vi "401_Add_AuditDataToDB.vi"(0 "Str(T)/Num":bool, 2 "Activity":string, 3 "Current Value":dbl, 4 "Previous Value":dbl, 5 "Activity":T2=enum."User show functionality for Info", 6 "Enum(F)/Str":bool, 7 "error in (no error)":errorcluster, 8 "Current Value":string, 12 "Previous Value":string) -> (27 "error out":errorcluster)   [LabVIEW 2015]
uses:
  Utilities/TypeDefs/401_Audit_Activity.ctl
  <vilib>/addons/database/Connection.llb/Conn ObjectReference.ctl
  System Settings/Modules/LV2GActions.ctl
  <vilib>/addons/database/NI_Database_API.lvlib
  <vilib>/addons/database/Connection.llb/DB Tools Open Connec (String).vi
panel:
  in  "Refnum in":T1
  out "Refnum out":T1
  # "INPUT"
  # "OUTPUT"
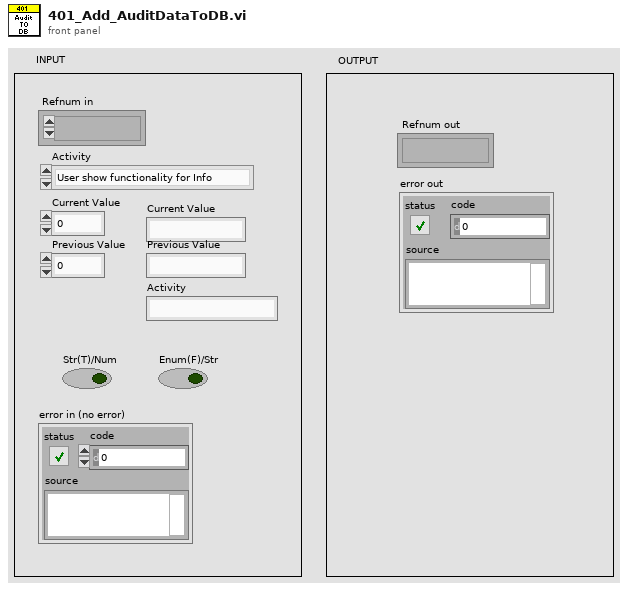
[diagram p1: front panel]
types:
  T1 = typedef "NI_Database_API.lvlib/Conn ObjectReference.ctl" = refnum<k1>
  T2 = typedef "401_Audit_Activity.ctl" = enum16{"User login sucessfully", "User login fail", "User lock", "User sign out", "User added succesfully", "User edit succesFully", "User delete succesfully", "Reset password", "Forgot Password", "User change security policy", "User change user rights", "User allowed functionality for inspection", "User allowed  functionality for recipe", "User allowed functionality for teach", "User allowed  for user management", "User allowed for camera settings", "User allowed functionality for Hardware Check", "User allowed functionality for printer settings", "User allowed functionality for server settings", "User allowed  for third party settings", "User allowed  for System settings", "User allowed functionality For Test I/O", "User allowed and show functionality For Fault Images", "User allowed functionality for Production Report", "User allowed functionality for Audit Report", "User allowed functionality for Help", "User allowed functionality for  Info", "User show functionality for Inspection", "User show functionality for Teach", "User show functionality for Recipe", "User show functionality for User Management", "User show functionality for Camera Settings", "User show functionality for Hardware Check", "User show functionality for printer Settings", "User show functionality  for Server Settings", "User show functionality for Third party Settings", "User show functionality for System settings", "User show functionality for Test I/O", "User show functionality for Fault Images", "User show functionality for Production Report", "User show functionality for Audit Report", "User show functionality for Help", "User show functionality for Info", "User update Security Policy", "User added Recipe sucessfully", "User delete Recipe sucessfully", "User rename Recipe sucessfully", "User save Camera Settings sucessfully ", "User Close with out save", "User change Brightness", "User change Exposure Time", "User change Gain Value", "User change Saturation", "User change Gamma", "User change Sharpness", "User change Hue", "User change White Balance", "User change  Comport ", "User save Test I/o settings sucessfully", "User close with out saving ", "User change Light Timing ", "User change Light Flash ", "Camera Ready", "User change Inactive Period ", "User change Grab Delay", "User change Timed Output", "User change No Of Track", "User change Output Polarity ", "User chnage Output Timing", "User change Track Output ", "User Taught sucessfully", "User close with out  Taught.", "User could not able To Add User", "User could not Delete", "User could not Updated", "User could not change Security Policy", "User could not change User Rights"}
  T3 = typedef "LV2GActions.ctl" = enum16{"Read", "Write", "Current", "Update", "UpdateSystemSettings", "UpdateModel"}
  T4 = cluster{"UserName":string, "Group Level":u16, "Theme":u16, "Software Type":u16, "System Language":u16, "Master":bool, "Recipe":string, "Batch":string, "Simulate":bool, "Trigger Activation":u16, "DateFormat":u16, "HardwareTest":bool}
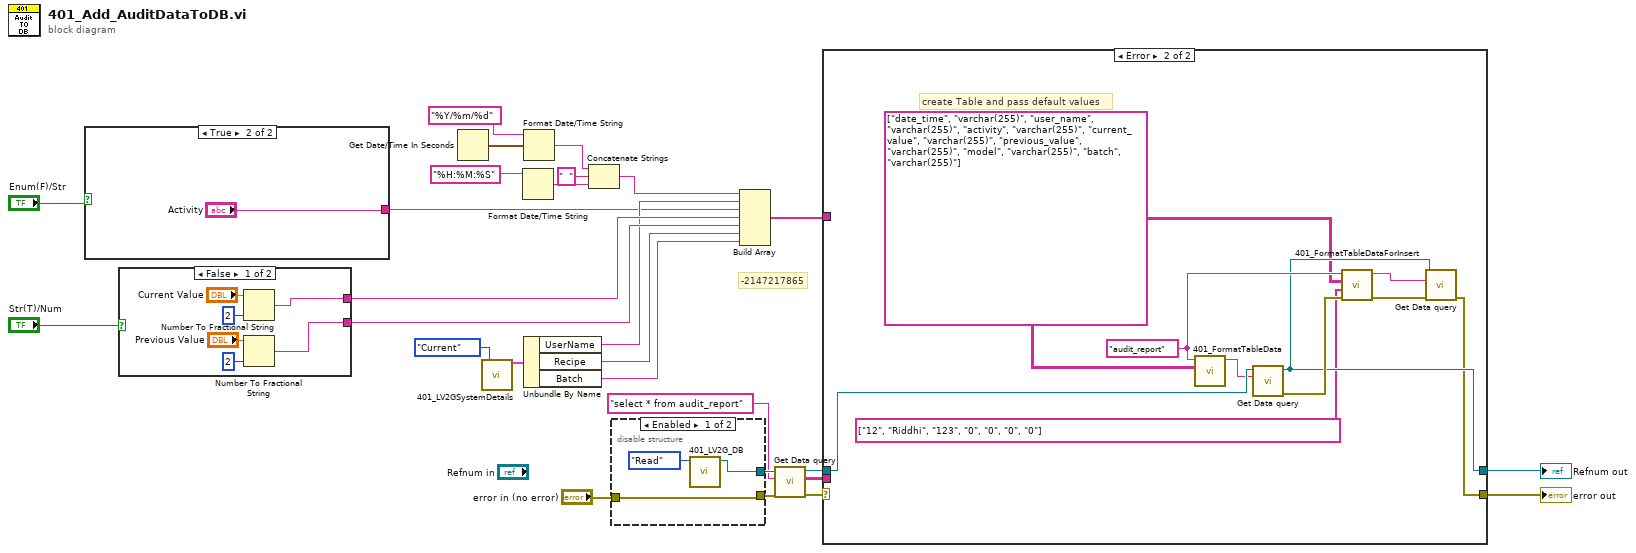
[diagram p0: block diagram]
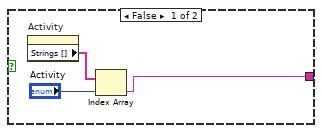
[diagram p2: hidden frame]
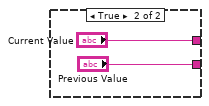
[diagram p3: hidden frame]
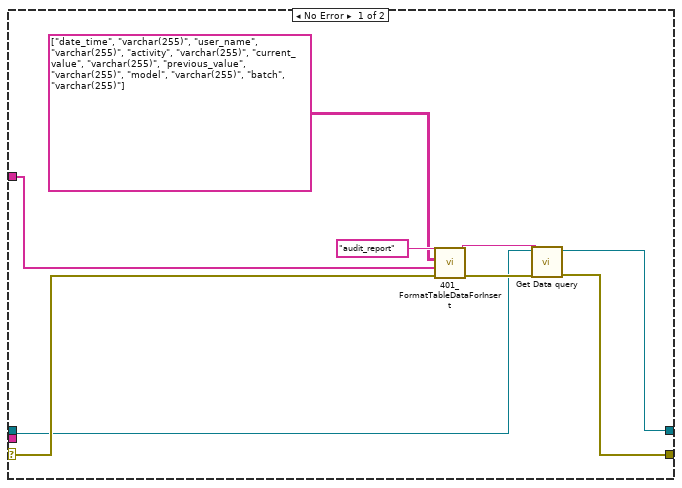
[diagram p4: hidden frame]
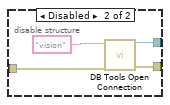
[diagram p5: hidden frame]
diagram:
  # "-2147217865"
  n1 = case shown="True" "Enum(F)/Str" {
    tunnel: [w30 "Activity"] -> w1
    frame False {
      n2 = property on="Activity" class="Enum (strict)"() -> ("Strings []"=w29:string[])  [unwired: 2 in, 2 out]
      n3 = Index Array(array=w29, index="Activity") -> (element=w30:string)
    }
    frame True {
    }
  }
  n4 = case shown="False" "Str(T)/Num" {
    tunnel: [w33 "Current Value"] -> w11
    tunnel: [w32 "Previous Value"] -> w10
    frame False {
      n5 = Number To Fractional String(number="Current Value", precision (6)=i16 2) -> (F-format string=w33:string)  [unwired: 2 in]
      n6 = Number To Fractional String(number="Previous Value", precision (6)=i16 2) -> (F-format string=w32:string)  [unwired: 2 in]
    }
    frame True {
    }
  }
  n7 = Get Date/Time In Seconds() -> (seconds since 1Jan1904=w16:timestamp)
  n8 = call "401_LV2GSystemDetails.vi"("R/W/C"=LV2GActions."Current") -> ("DataOut"=w9:T4)  [unwired: 17 in, 1 out]
  n9 = Format Date/Time String(time format string (%c)="%H:%M:%S") -> (date/time string=w14:string)  [unwired: 2 in]
  n10 = Format Date/Time String(time format string (%c)="%Y/%m/%d" ("format string"), seconds (now)=w16) -> (date/time string=w19:string)  [unwired: 1 in]
  n11 = Unbundle By Name(w9) -> ("UserName"=w7:string, "Recipe"=w6:string, "Batch"=w5:string)
  n12 = Concatenate Strings(w19, "  " ("string"), w14) -> (w15:string)
  n13 = disable-structure shown="Enabled" {
    disable-tunnel: [w42 w44] -> w26
    disable-tunnel: [w40 w45] -> w22
    disable-tunnel: "error in (no error)" -> [w42 w43]
    frame Enabled {
      n14 = call "401_LV2G_DB.vi"("Action"=enum16{"Open", "Read", "Close"}."Read") -> ("DB_Ref"=w40:T1)  [unwired: 9 in, 1 out]
    }
    frame Disabled {
      n15 = call-poly <vilib>:"DB Tools Open Connection.vi"("error in (no error)"=w43, "connection information"="vision" ("userID")) -> ("error out"=w44:errorcluster, "connection reference"=w45:T1)  [unwired: 6 in]
    }
  }
  n16 = Build Array(w15, w7, w1, w11, w10, w6, w5) -> (w13:string[])
  n17 = call "Get Data query.vi"("error in"=w26, "SQL query"="select * from audit_report", "connection reference"=w22) -> ("error Out"=w25:errorcluster, "Data_Table"=w27:string[][], "connection reference"=w24:T1)  [unwired: 6 in]
  n18 = case shown="Error" w25 {
    selector: w25 -> [w53 _]
    tunnel: w27 -> [_ _]
    tunnel: w24 -> [w51 w65]
    tunnel: [w50 w62] -> w23
    tunnel: [w47 w56] -> w21
    tunnel: w13 -> [w54 _]
    frame No Error {
      n19 = call "401_FormatTableDataForInsert.vi"("Error In"=w53, "Values"=w54, "ColoumnNames+DataType"=string[][] [["date_time", "varchar(255)"], ["user_name", "varchar(255)"], ["activity", "varchar(255)"], ["current_value", "varchar(255)"], ["previous_value", "varchar(255)"], ["model", "varchar(255)"], ["batch", "varchar(255)"]], "Table_Name"="audit_report") -> ("ErrorOut"=w52:errorcluster, "Query"=w48:string)  [unwired: 6 in]
      n20 = call "Get Data query.vi"("error in"=w52, "SQL query"=w48, "connection reference"=w51) -> ("error Out"=w47:errorcluster, "connection reference"=w50:T1)  [unwired: 6 in, 1 out]
    }
    frame Error {
      w59 = string[][] [["date_time", "varchar(255)"], ["user_name", "varchar(255)"], ["activity", "varchar(255)"], ["current_value", "varchar(255)"], ["previous_value", "varchar(255)"], ["model", "varchar(255)"], ["batch", "varchar(255)"]] ("ColoumnNames+DataType")
      w64 = "audit_report" ("Table_Name")
      # "create Table and pass default values"
      n21 = call "401_FormatTableData.vi"("ColoumnNames+DataType"=w59, "Table_Name"=w64) -> ("Query"=w57:string)  [unwired: 9 in]
      n22 = call "Get Data query.vi"("SQL query"=w57, "connection reference"=w65) -> ("error Out"=w63:errorcluster, "connection reference"=w62:T1)  [unwired: 7 in, 1 out]
      n23 = call "401_FormatTableDataForInsert.vi"("Error In"=w63, "Values"=string[] ["12", "Riddhi", "123", "0", "0", "0", "0"], "ColoumnNames+DataType"=w59, "Table_Name"=w64) -> ("ErrorOut"=w61:errorcluster, "Query"=w58:string)  [unwired: 6 in]
      n24 = call "Get Data query.vi"("error in"=w61, "SQL query"=w58, "connection reference"=w62) -> ("error Out"=w56:errorcluster)  [unwired: 6 in, 2 out]
    }
  }
  "error out" <- w21
  "Refnum out" <- w23
